vi "General-InsertContrastInFile.vi"(0 "refnum IN":refnum<file>, 1 "tiempo (ms)":u32, 2 "contraste":dbl, 3 "error IN":errorcluster, 4 "Status":string) -> (5 "refnum OUT":refnum<file>, 6 "error OUT":errorcluster)   [LabVIEW 2010]
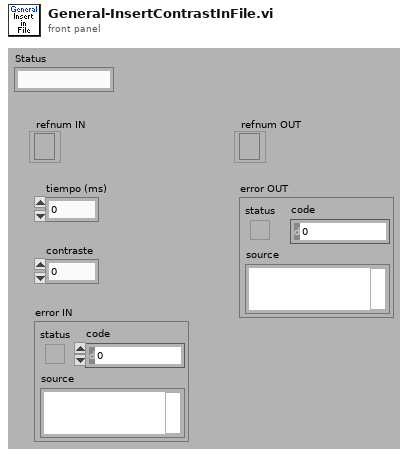
[diagram p1: front panel]
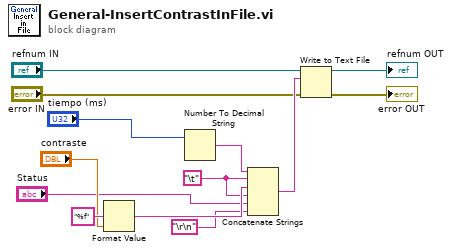
[diagram p0: block diagram]
diagram:
  w2 = "\t"
  n1 = Format Value(format string="%f", value (0)="contraste") -> (output string=w12:string)  [unwired: 1 in]
  n2 = Number To Decimal String(number="tiempo (ms)") -> (decimal integer string=w9:string)  [unwired: 1 in]
  n3 = Concatenate Strings(w9, w2, w12, w2, "Status", "\r\n") -> (w10:string)
  n4 = Write to Text File(file (use dialog)="refnum IN", text=w10, error in="error IN") -> (refnum out=→"refnum OUT":refnum<file>, error out=→"error OUT":errorcluster)  [unwired: 1 in, 1 out]
